vi "NoErrorConstant.vi"() -> (1 "error out (no Error)":errorcluster)   [LabVIEW 2021]
doc: "Enthält nichts anderes als eine Konstante \"no Error\".\nWird aus kosmetischen Gründen benutzt, da dieses VI optisch nicht so viel Fläche im Diagramm beansprucht wie eine Konstante"
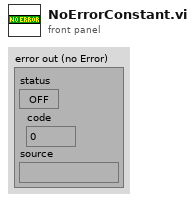
[diagram p1: front panel]
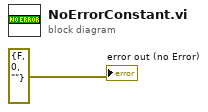
[diagram p0: block diagram]
diagram:
  "error out (no Error)" <- errorcluster {"status"=FALSE, "code"=0, "source"=""} ("error in")
